vi "Prueba1.vi"() -> ()   [LabVIEW 2020]
uses:
  Libraries/Osciloscope/Osciloscope.lvlib
panel:
  out "error out":errorcluster
  out "Osciloscopes":string[](array[string])
  out "Waveform Graph":waveform(dbl)(graph)
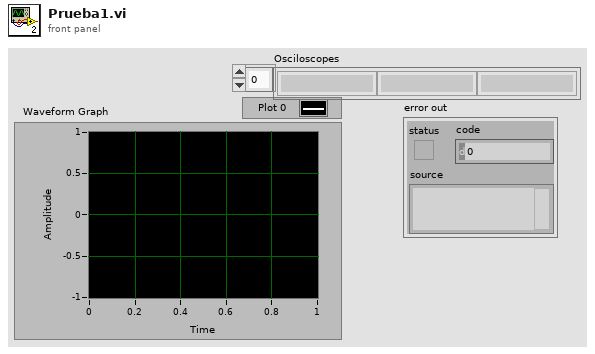
[diagram p1: front panel]
types:
  T1 = typedef "Osciloscope.lvlib/Broadcast Events--cluster.ctl" = cluster{"Module Did Init":refnum<user-event>, "Status Updated":refnum<user-event>, "Error Reported":refnum<user-event>, "Module Did Stop":refnum<user-event>, "Update Module Execution Status":refnum<user-event>, "OsciloscopesTypes":refnum<user-event>}
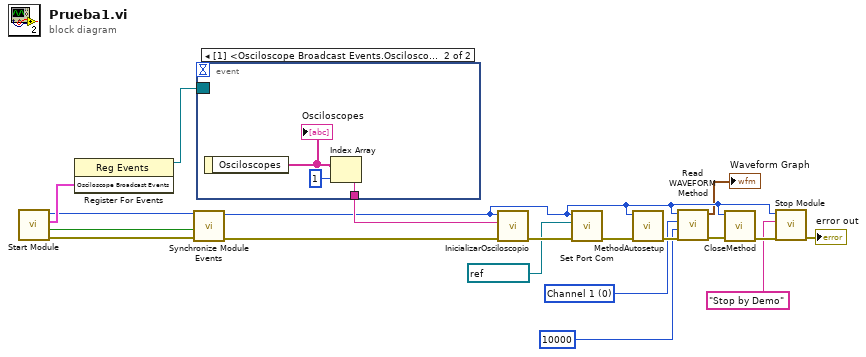
[diagram p0: block diagram]
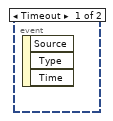
[diagram p2: hidden frame]
diagram:
  w6 = u16 0 items=["Channel 1", "Channel 2", "Channel 3", "Channel 4", "Math", "Reference A", "Reference B", "Reference C", "Reference D", "FFT"] ("Source (0: Channel 1)")
  n1 = call "Start Module.vi"() -> ("error out"=w15:errorcluster, "Wait for Event Sync?"=w3:bool, "Osciloscope Broadcast Events"=w19:T1, "Module ID"=w18:i32)  [unwired: 8 in]
  n2 = register-events(w19) -> (reference out=w17:refnum<event-registration>)  [unwired: 2 in, 1 out]
  n3 = call "Synchronize Module Events.vi"("error in"=w15, "Wait for Event Sync?"=w3, "Module ID in"=w18) -> ("error out"=w14:errorcluster, "Module ID out"=w7:i32)  [unwired: 7 in]
  n4 = event shown="[1] <Osciloscope Broadcast Events.OsciloscopesTypes>: User Event" {
    selector: w17 -> [_ _]
    dyn-events: _ -> [_ _]
    timeout: _ -> [_ _]
    tunnel: [_ w21] -> w16
    event Timeout {
      n5 = event-data() -> ()  [unwired: 1 in, 3 out]
    }
    event User Event {
      n6 = event-data() -> ("Osciloscopes"=w22:string[])  [unwired: 1 in]
      "Osciloscopes" <- w22
      n7 = Index Array(array=w22, index=1) -> (element=w21:string)
    }
  }
  n8 = call "InicializarOsciloscopio.vi"("error in"=w14, "OsciloscopioName"=w16, "Module ID"=w7) -> ("error out"=w13:errorcluster)  [unwired: 8 in]
  n9 = call "Set Port Com.vi"("error in"=w13, "COM"=refnum<visa-resource-name> "COM2", "Module ID"=w7) -> ("error out"=w11:errorcluster)  [unwired: 8 in]
  n10 = call "MethodAutosetup.vi"("error in"=w11, "Module ID"=w7) -> ("error out"=w10:errorcluster)  [unwired: 9 in]
  n11 = call "Read WAVEFORM Method.vi"("error in"=w10, "Timeout (10000 ms)"=u32 10000, "Source (0: Channel 1)"=w6, "Module ID"=w7) -> ("error out"=w9:errorcluster, "Waveform Data"=→"Waveform Graph":waveform(dbl))  [unwired: 5 in, 1 out]
  n12 = call "CloseMethod.vi"("error in"=w9, "Module ID"=w7) -> ("error out"=w8:errorcluster)  [unwired: 9 in]
  n13 = call "Stop Module.vi"("error in (no error)"=w8, "Origin"="Stop by Demo", "Module ID"=w7) -> ("error out"=→"error out":errorcluster)  [unwired: 8 in]
